vi "Chamber_control_Aug_ 2018.vi"() -> ()   [LabVIEW 2014]
doc: "This template is for the Queued Message Handler design pattern.\n\nThe Event Handling Loop generates messages based on user interface actions.\n\nThe Message Handling Loop processes messages generated by the Event Handling Loop, or by other messages. The messages are string values, so new messages can be added easily to the Message Cases case structure in the Message Handling Loop. Each message cluster can also provide an optional value for Message Data, which is a variant that can be converted to whatever message-specific data is required."
uses:
  <vilib>/Analysis/baseanly.llb/Mean (DBL).vi
  <vilib>/Instr/_visa.llb/VISA Configure Serial Port (Instr).vi
  Environmental Chamber LabVIEW and Instruments/Drivers and Software/Keithley 2100 Series/Public/Configure/Configure 2 Wire Resistance.vi
  <vilib>/Utility/file.llb/Read From Spreadsheet File (string).vi
  <vilib>/Utility/file.llb/Write To Spreadsheet File (string).vi
  Environmental Chamber LabVIEW and Instruments/Drivers and Software/LabVIEW 8.2 Drivers/keithley_24xx/Keithley 24XX/Public/Data/Read (Single Point).vi
  Environmental Chamber LabVIEW and Instruments/Drivers and Software/keithley_6430/Keithley 6430/Public/Data/Read (Single Point).vi
  Environmental Chamber LabVIEW and Instruments/Drivers and Software/keithley_6430/Keithley 6430/Keithley 6430.lvlib
  Environmental Chamber LabVIEW and Instruments/Drivers and Software/Keithley 2100 Series/Keithley 2100 Series.lvlib
  Environmental Chamber LabVIEW and Instruments/Drivers and Software/keithley_24xx/Keithley 24XX/Keithley 24XX.lvlib
  <vilib>/Analysis/NI_AALBase.lvlib
panel:
  in  "K2420 DC bias (V)":dbl=0.05
  in  "SYSTEM CONTROL":T1={"valve % open"=0.0, "Desired pressure"=0.0, "set Vapor sccm"=0.0, "set Gas sccm"=0.0, "Valve mode"=enum."% Open", "Pressure Mode"=enum."Abs. pressure", "analyte partial pressure"=23.8, "Actual"=0.0, "Read pressure (Torr)"=0.0, "Read vapor flow (sccm)"=0.0, "Read gas flow (sccm)"=0.0, "Save now"=FALSE, "Stop after seq."=TRUE, "Turbo pump\nauto on"=TRUE, "Integrate points"=0} caption="Pressure settings" {"Integrate points" min=0 max=100 step=1; "analyte partial pressure" min=0.0 max=100.0 step=5.0; "set Gas sccm" min=0 max=200 step=5; "set Vapor sccm" min=0 max=200 step=5; "Desired pressure" min=0.0 max=760.0 step=5.0; "valve % open" min=0.0 max=100.0 step=5.0 format="%#_2f"}
  in  "SAVE SAMPLE / ANALYTE NAMES":T2={"QCM1"="", "QCM2"="", "QCM3"="", "QCM4"="broken", "QCM5"="NOT WORKING", "QCM6"="", "SRS"="bareAu", "K-2420"="", "K-6430"="", "K-2100"="", "Gas"="NOT WORKING", "Vapor"="H2O", "Notes"=""} caption="Save samplffe names"
  in  "Clear all charts":bool
  out "K-6430":dbl(graph)
  out "K-2420":dbl(graph)
  out "File":path caption="DATA FILE"
  in  "Stop":bool
  out "QCM plot":T3(graph)
  out "K-2100":dbl(graph)
  out "State date/time":string caption="Program start time"
  out "J-KEM temp":dbl(graph)
  out "saving data?":bool
  out "pressure chart":dbl(graph)
  in  "SEQUENCE":T4 {"preview" items=["pressure", "gas flow", "vapor flow", "bias"]}
  # "100"
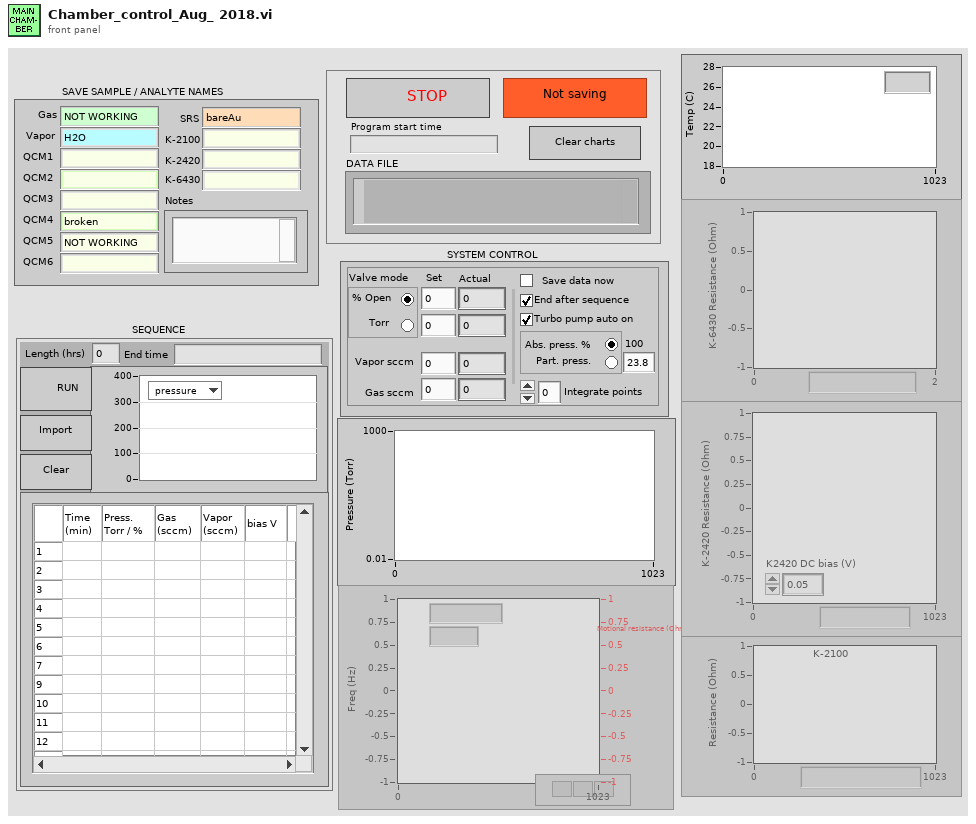
[diagram p1: front panel]
types:
  T1 = cluster{"valve % open":dbl, "Desired pressure":dbl, "set Vapor sccm":sgl, "set Gas sccm":sgl, "Valve mode":enum32{"% Open", "Torr "}, "Pressure Mode":enum32{"Abs. pressure", " Part. pressure"}, "analyte partial pressure":dbl, "Actual":dbl, "Read pressure (Torr)":dbl, "Read vapor flow (sccm)":dbl, "Read gas flow (sccm)":dbl, "Save now":bool, "Stop after seq.":bool, "Turbo pump\nauto on":bool, "Integrate points":i32}
  T2 = cluster{"QCM1":string, "QCM2":string, "QCM3":string, "QCM4":string, "QCM5":string, "QCM6":string, "SRS":string, "K-2420":string, "K-6430":string, "K-2100":string, "Gas":string, "Vapor":string, "Notes":string}
  T3 = cluster{"Frequency out":dbl, "Resistance out":dbl}
  T4 = cluster{"Run Sequence":bool, "User-defined\nsequence":string[][], "preview":u16, "Sequence\npreview":cluster{dbl[], dbl[]}[], "Clear sequence":bool, "Import sequence file":bool, "Length (hrs)":dbl, "End time":string}
  T5 = cluster{"Keithley 6430":bool, "J-KEM":bool, "Keithley 2420":bool, "Keithley 2100":bool, "SRS QCM":bool, "Pressure control":bool, "Arduino":bool}
  T6 = enum16{"open", "replace", "create", "open or create", "replace or create", "replace or create with confirmation"}
  T7 = enum8{"Enabled", "Disabled", "Disabled and Grayed Out"}
  T8 = cluster{"Frequency out":dbl, "Resistance out":dbl}[]
  T9 = cluster{"VISA resource name":refnum<visa-resource-name>, "error out":errorcluster, bool}
  T10 = cluster{"VISA resource name out":refnum<visa-resource-name>, "error out":errorcluster, bool}
  T11 = cluster{bool, "task out":refnum<k21>, "error out":errorcluster, "task out":refnum<k21>, "error out":errorcluster, "turbo pump":refnum<visa-resource-name>, "error out":errorcluster}
  T12 = cluster{bool, "task out":refnum<k21>, "error out":errorcluster, "task out":refnum<k21>, "error out":errorcluster, "VISA resource name out":refnum<visa-resource-name>, "error out":errorcluster}
  T13 = cluster{bool, "VISA resource name":refnum<visa-resource-name>, "error out":errorcluster}
  T14 = cluster{bool, "VISA resource name out":refnum<visa-resource-name>, "error out":errorcluster}
  T15 = cluster{bool, "VISA in":refnum<visa-resource-name>, "error out":errorcluster}
  T16 = cluster{bool, "VISA out":refnum<visa-resource-name>, "error out":errorcluster}
  T17 = cluster{"[0]":string, "[1]":string, "[2]":string, "[3]":string, "[4]":string, "[5]":string}
  T18 = cluster{string[][], path, "data headers":string[]}
  T19 = cluster{"Boolean":bool, "VISA resource name out":refnum<visa-resource-name>, "error out":errorcluster}
  T20 = cluster{"Boolean":bool, "VISA out":refnum<visa-resource-name>, "error out":errorcluster}
  T21 = cluster{cluster{bool, "VISA resource name out":refnum<visa-resource-name>, "error out":errorcluster}, "Address out":cluster{"Boolean":bool, "VISA resource name out":refnum<visa-resource-name>, "error out":errorcluster}, cluster{bool, "VISA resource name out":refnum<visa-resource-name>, "error out":errorcluster}, cluster{bool, "VISA resource name out":refnum<visa-resource-name>, "error out":errorcluster}, "SRS address out":cluster{"Boolean":bool, "VISA out":refnum<visa-resource-name>, "error out":errorcluster}}
  T22 = cluster{"valve % open":dbl, "Desired pressure":dbl, "set Vapor sccm":sgl, "set Gas sccm":sgl, "Valve mode":enum32{"% Open", "Torr "}, "Pressure Mode":enum32{"Abs. pressure", " Part. pressure"}, "analyte partial pressure":dbl}
  T23 = cluster{"User-defined\nsequence":string[][], "Present (s)":dbl, "current  step # in":i32, "sequence end time in":timestamp}
  T24 = cluster{"current  step # in":i32, "sequence end time in":timestamp, "Boolean":bool}
  T25 = cluster{"press/RH/gas/vapor":cluster{"pressure":string, "RH":string, "gas flow":string, "vapor flow":string}, "Cluster":cluster{"Valve position (%)":dbl, "read pressure":dbl, "read vapor flow":dbl, "read gas flow":dbl}}
  T26 = cluster{"Boolean":bool, "task out":refnum<k21>, "error out":errorcluster, "task out":refnum<k21>, "error out":errorcluster, "VISA resource name out":refnum<visa-resource-name>, "error out":errorcluster}
  T27 = cluster{"t":string, "delta t":string, "p":string, "delta p":string}
  T28 = cluster{"pressure":string, "RH":string, "gas flow":string, "vapor flow":string}
  T29 = cluster{"Valve position (%)":dbl, "read pressure":dbl, "read vapor flow":dbl, "read gas flow":dbl}
  T30 = cluster{"[0]":dbl, "[1]":dbl, "[2]":dbl, "[3]":dbl, "[4]":dbl, "[5]":dbl}[]
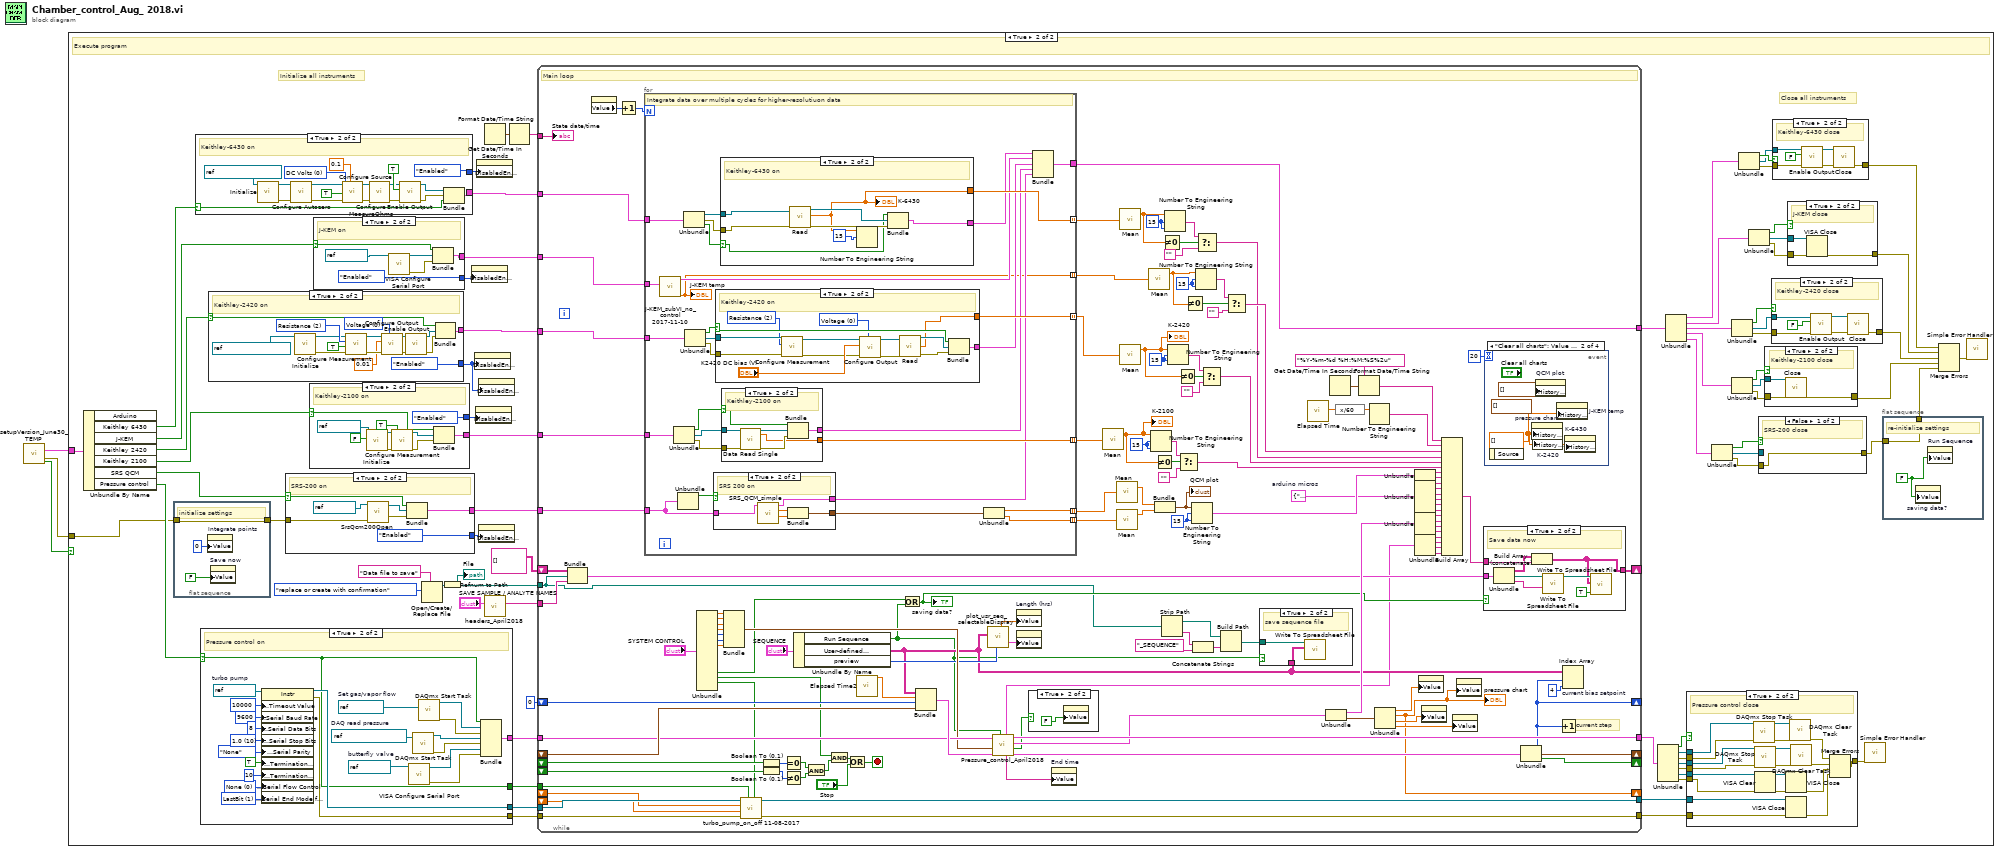
[diagram p0: block diagram]
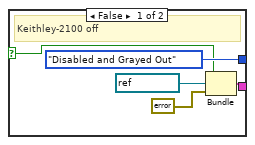
[diagram p4: hidden frame]
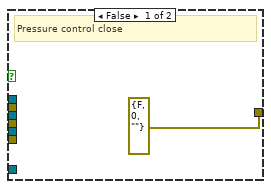
[diagram p5: hidden frame]
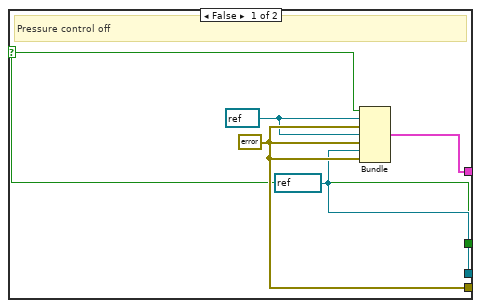
[diagram p6: hidden frame]
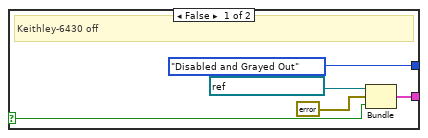
[diagram p8: hidden frame]
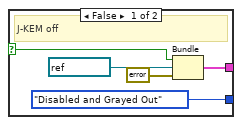
[diagram p10: hidden frame]
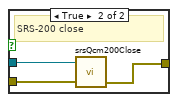
[diagram p11: hidden frame]
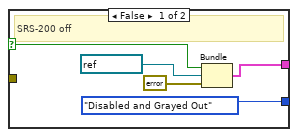
[diagram p12: hidden frame]
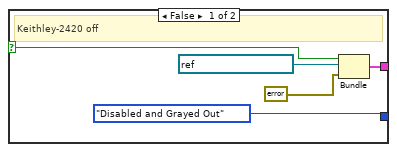
[diagram p14: hidden frame]
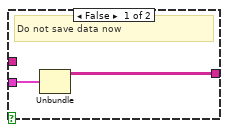
[diagram p16: hidden frame]
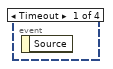
[diagram p17: hidden frame]
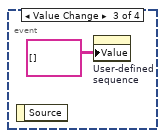
[diagram p18: hidden frame]
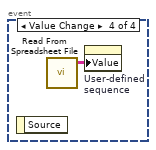
[diagram p19: hidden frame]
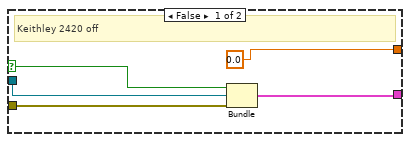
[diagram p20: hidden frame]
diagram:
  n1 = call "setupVersion_June30_TEMP.vi"() -> ("Instruments on/off"=w1:T5, "error IO"=w2:errorcluster, "OK"=w3:bool)  [unwired: 13 in]
  n2 = case shown="True" w3 {
    tunnel: w2 -> [_ w44]
    tunnel: w1 -> [_ w51]
    frame False {
      # "Cancel program"
    }
    frame True {
      # "Close all instruments"
      # "Initialize all instruments"
      # "Execute program"
      n3 = Unbundle By Name(w51) -> ("Keithley 6430"=w50:bool, "J-KEM"=w49:bool, "Keithley 2420"=w48:bool, "Keithley 2100"=w47:bool, "SRS QCM"=w46:bool, "Pressure control"=w45:bool)  [unwired: 1 out]
      n4 = flat-sequence {
        tunnel: [w78] -> w43
        tunnel: w44 -> [w78]
        frame #0 {
          # "initialize settings"
          n5 = property on="Integrate points" class="DigNum (strict)"("Value"=0) -> ()  [unwired: 2 in, 2 out]
          n6 = property on="Save now" class="Bool (strict)"("Value"=FALSE) -> ()  [unwired: 2 in, 2 out]
        }
      }
      n7 = case shown="True" w50 {
        selector: w50 -> [w156 w176]
        tunnel: [T7."Disabled and Grayed Out" ("Disabled") T7."Enabled" ("Disabled")] -> w30
        tunnel: [w155 w175] -> w28
        frame False {
          # "Keithley-6430 off"
          n8 = Bundle("VISA resource name"=refnum<visa-resource-name> "GPIB0::29::INSTR", "error out"=errorcluster {"status"=FALSE, "code"=0, "source"=""}, w156) -> (w155:T9)  [unwired: 1 in]
        }
        frame True {
          w163 = u16 0 items=["DC Volts", "DC Current"] ("Source Function (0: DC Volts)")
          # "Keithley-6430 on"
          n9 = call "Initialize.vi"("VISA resource name"=refnum<visa-resource-name> "GPIB2::19::INSTR") -> ("error out"=w169:errorcluster, "VISA resource name out"=w170:refnum<visa-resource-name>)  [unwired: 4 in, 5 out]
          n10 = call "Configure Autozero.vi"("error in (no error)"=w169, "VISA resource name"=w170) -> ("error out"=w166:errorcluster, "VISA resource name out"=w168:refnum<visa-resource-name>)  [unwired: 8 in]
          n11 = call "Configure Source.vi"("V-Source Level [V]"=0.1, "error in (no error)"=w166, "Auto Range (T:Enable)"=TRUE, "Source Function (0: DC Volts)"=w163, "VISA resource name"=w168) -> ("error out"=w165:errorcluster, "VISA resource name out"=w167:refnum<visa-resource-name>)  [unwired: 5 in]
          n12 = call "Configure MeasureOhms.vi"("error in (no error)"=w165, "VISA resource name"=w167) -> ("error out"=w174:errorcluster, "VISA resource name out"=w172:refnum<visa-resource-name>)  [unwired: 4 in, 4 out]
          n13 = call "Enable Output.vi"("error in (no error)"=w174, "Enable Output (F:Off)"=TRUE ("Output (F:Off)"), "VISA resource name"=w172) -> ("error out"=w161:errorcluster, "VISA resource name out"=w162:refnum<visa-resource-name>)  [unwired: 7 out]
          n14 = Bundle("VISA resource name out"=w162, "error out"=w161, w176) -> (w175:T10)  [unwired: 1 in]
        }
      }
      n15 = case shown="True" w45 {
        selector: w45 -> [w120 w126]
        tunnel: [w124 w127] -> w42
        tunnel: [w123 w125] -> w34
        tunnel: [w121 w128] -> w35
        tunnel: [w120 w126] -> w33
        frame False {
          w121 = refnum<visa-resource-name> refnum ("turbo pump")
          w122 = refnum<k21> refnum ("task out")
          w123 = errorcluster {"status"=FALSE, "code"=0, "source"=""} ("error out")
          # "Pressure control off"
          n16 = Bundle(w120, "task out"=w122, "error out"=w123, "task out"=w122, "error out"=w123, "turbo pump"=w121, "error out"=w123) -> (w124:T11)  [unwired: 1 in]
        }
        frame True {
          w132 = u16 1 items=["None", "LastBit", "TermChar"] ("Serial Settings:Serial End Mode for Reads")
          w130 = u16 0 items=["None", "XON/XOFF", "RTS/CTS", "XON/XOFF & RTS/CTS", "DTR/DSR", "XON/XOFF & DTR/DSR"] ("flow control (0:none)")
          w133 = u16 10 items=["1.0"=10, "1.5"=15, "2.0"=20] ("stop bits (10: 1 bit)")
          w129 = refnum<visa-resource-name> "COM7"  # turbo pump
          w145 = refnum<visa-resource-name> "COM5"  # butterfly valve
          w146 = refnum<k21> "Setflow"  # Set gas/vapor flow
          w147 = refnum<k21> "AllDaqReadings"  # DAQ read pressure
          # "Pressure control on"
          n17 = property class="Instr"(reference=w129, "General Settings:Timeout Value"=u32 10000 ("timeout (10sec)"), "Serial Settings:Serial Baud Rate"=u32 9600 ("baud rate (9600)"), "Serial Settings:Serial Data Bits"=u16 8 ("data bits (8)"), "Serial Settings:Serial Stop Bits"=w133, "Serial Settings:Serial Parity"=enum16{"None", "Odd", "Even", "Mark", "Space"}."None" ("parity (0:none)"), "Message Based Settings:Termination Character Enable"=TRUE ("Enable Termination\nChar (T)"), "Message Based Settings:Termination Character"=u8 10 ("termination char\n(0xA = '\\n' = LF)"), "Serial Settings:Serial Flow Control"=w130, "Serial Settings:Serial End Mode for Reads"=w132) -> (reference out=w128:refnum<visa-resource-name>, error out=w125:errorcluster)  [unwired: 1 in]
          n18 = call-poly "VISA Configure Serial Port"("VISA resource name"=w145) -> ("VISA resource name out"=w140:refnum<visa-resource-name>, "error out"=w139:errorcluster)  [unwired: 13 in]
          n19 = call <vilib>:"DAQmx Start Task.vi"("task/channels in"=w147) -> ("task out"=w142:refnum<k21>, "error out"=w141:errorcluster)  [unwired: 13 in]
          n20 = call <vilib>:"DAQmx Start Task.vi"("task/channels in"=w146) -> ("task out"=w144:refnum<k21>, "error out"=w143:errorcluster)  [unwired: 13 in]
          n21 = Bundle(w126, "task out"=w144, "error out"=w143, "task out"=w142, "error out"=w141, "VISA resource name out"=w140, "error out"=w139) -> (w127:T12)  [unwired: 1 in]
        }
      }
      n22 = case shown="True" w48 {
        selector: w48 -> [w219 w224]
        tunnel: [T7."Disabled and Grayed Out" ("Disabled") T7."Enabled" ("Disabled")] -> w17
        tunnel: [w217 w221] -> w27
        frame False {
          # "Keithley-2420 off"
          n23 = Bundle(w219, "VISA resource name"=refnum<visa-resource-name> "GPIB1::24::INSTR", "error out"=errorcluster {"status"=FALSE, "code"=0, "source"=""}) -> (w217:T13)  [unwired: 1 in]
        }
        frame True {
          w230 = u16 0 items=["Voltage", "Current"] ("Source Mode  (0: Voltage)")
          w235 = u16 2 items=["Volts", "Current", "Resistance"] ("Function (0: Volts)")
          # "Keithley-2420 on"
          n24 = call "Initialize.vi"("VISA resource name"=refnum<visa-resource-name> "GPIB1::24::INSTR") -> ("error out"=w225:errorcluster, "VISA resource name out"=w226:refnum<visa-resource-name>)  [unwired: 9 in]
          n25 = call "Configure Measurement.vi"("error in (no error)"=w225, "Enable Auto Range (T:Enable)"=TRUE, "Function (0: Volts)"=w235, "VISA resource name"=w226) -> ("error out"=w234:errorcluster, "VISA resource name out"=w233:refnum<visa-resource-name>)  [unwired: 6 in]
          n26 = call "Configure Output.vi"("Source Mode  (0: Voltage)"=w230, "error in (no error)"=w234, "Output Level (0)"=0.01 ("K2420 Applied Voltage (V) 2"), "VISA resource name"=w233) -> ("error out"=w232:errorcluster, "VISA resource name out"=w231:refnum<visa-resource-name>)  [unwired: 6 in]
          n27 = call "Enable Output.vi"("error in (no error)"=w232, "VISA resource name"=w231) -> ("error out"=w222:errorcluster, "VISA resource name out"=w223:refnum<visa-resource-name>)  [unwired: 8 in]
          n28 = Bundle(w224, "VISA resource name out"=w223, "error out"=w222) -> (w221:T14)  [unwired: 1 in]
        }
      }
      n29 = case shown="True" w46 {
        selector: w46 -> [w198 w204]
        tunnel: w43 -> [_ w207]
        tunnel: [T7."Disabled and Grayed Out" ("Disabled") T7."Enabled" ("Disabled")] -> w59
        tunnel: [w197 w203] -> w25
        frame False {
          # "SRS-200 off"
          n30 = Bundle(w198, "VISA in"=refnum<visa-resource-name> "COM6", "error out"=errorcluster {"status"=FALSE, "code"=0, "source"=""}) -> (w197:T15)  [unwired: 1 in]
        }
        frame True {
          # "SRS-200 on"
          n31 = call "SrsQcm200Open.vi"("error in"=w207, "VISA in"=refnum<visa-resource-name> "COM6") -> ("error out"=w202:errorcluster, "VISA out"=w205:refnum<visa-resource-name>)  [unwired: 3 in]
          n32 = Bundle(w204, "VISA out"=w205, "error out"=w202) -> (w203:T16)  [unwired: 1 in]
        }
      }
      n33 = case shown="True" w47 {
        selector: w47 -> [w88 w92]
        tunnel: [T7."Disabled and Grayed Out" ("Disabled") T7."Enabled" ("Disabled")] -> w57
        tunnel: [w85 w93] -> w26
        frame False {
          # "Keithley-2100 off"
          n34 = Bundle(w88, "VISA resource name out"=refnum<visa-resource-name> "K-2100", "error out"=errorcluster {"status"=FALSE, "code"=0, "source"=""}) -> (w85:T14)  [unwired: 1 in]
        }
        frame True {
          # "Keithley-2100 on"
          n35 = call "Initialize.vi"("VISA resource name"=refnum<visa-resource-name> "K-2100", "Reset? (T: Reset)"=FALSE) -> ("VISA resource name out"=w97:refnum<visa-resource-name>, "error out"=w96:errorcluster)  [unwired: 16 in]
          n36 = call-poly "Configure Measurement.vi"("VISA resource name"=w97, "error in (no error)"=w96, "Auto Range? (T: Auto)"=TRUE) -> ("VISA resource name out"=w91:refnum<visa-resource-name>, "error out"=w90:errorcluster)  [unwired: 15 in]
          n37 = Bundle(w92, "VISA resource name out"=w91, "error out"=w90) -> (w93:T14)  [unwired: 1 in]
        }
      }
      n38 = case shown="True" w49 {
        selector: w49 -> [w183 w189]
        tunnel: [w184 w190] -> w68
        tunnel: [T7."Disabled and Grayed Out" ("Disabled") T7."Enabled" ("Disabled")] -> w29
        frame False {
          # "J-KEM off"
          n39 = Bundle(w183, "VISA resource name"=refnum<visa-resource-name> "COM3", "error out"=errorcluster {"status"=FALSE, "code"=0, "source"=""}) -> (w184:T13)  [unwired: 1 in]
        }
        frame True {
          # "J-KEM on"
          n40 = call-poly "VISA Configure Serial Port"("VISA resource name"=refnum<visa-resource-name> "COM3") -> ("VISA resource name out"=w191:refnum<visa-resource-name>, "error out"=w188:errorcluster)  [unwired: 13 in]
          n41 = Bundle(w189, "VISA resource name out"=w191, "error out"=w188) -> (w190:T14)  [unwired: 1 in]
        }
      }
      n42 = Open/Create/Replace File(prompt="Data file to save", operation (0:open)=T6."replace or create with confirmation") -> (refnum out=w15:refnum<file>)  [unwired: 4 in, 2 out]
      n43 = Refnum to Path(1:w15) -> (0:w11:path)
      "File" <- w11
      n44 = property on="J-KEM temp" class="WFChart (strict)"("DisabledEnum"=w29) -> ()  [unwired: 2 in, 2 out]
      n45 = property on="K-2420" class="WFChart (strict)"("DisabledEnum"=w17) -> ()  [unwired: 2 in, 2 out]
      n46 = property on="K-2100" class="WFChart (strict)"("DisabledEnum"=w57) -> ()  [unwired: 2 in, 2 out]
      n47 = property on="K-6430" class="WFChart (strict)"("DisabledEnum"=w30) -> ()  [unwired: 2 in, 2 out]
      n48 = property on="K2420 DC bias (V)" class="DigNum (strict)"("DisabledEnum"=w17) -> ()  [unwired: 2 in, 2 out]
      n49 = property on="QCM plot" class="WFChart (strict)"("DisabledEnum"=w59) -> ()  [unwired: 2 in, 2 out]
      n50 = call "headers_April2018.vi"("Sample names"="SAVE SAMPLE / ANALYTE NAMES") -> ("data headers"=w10:string[])  [unwired: 10 in]
      n51 = Get Date/Time In Seconds() -> (seconds since 1Jan1904=w18:timestamp)
      n52 = Format Date/Time String(seconds (now)=w18) -> (date/time string=w56:string)  [unwired: 2 in]
      n53 = while {
        tunnel: w68 -> [w371]
        tunnel: w11 -> [w278]
        tunnel: w56 -> [w357]
        tunnel: w42 -> [w345]
        shift-right: [w332] -> _
        shift-left: 0 ("1st step") -> [w349]
        shift-right: [w354] -> _
        shift-left: _ -> [w352]
        shift-right: [w353] -> _
        shift-left: _ -> [w351]
        shift-left: _ -> [w350]
        tunnel: [w348] -> w53
        tunnel: w35 -> [w344]
        tunnel: w34 -> [w343]
        tunnel: w33 -> [w335]
        tunnel: [w341] -> w32
        tunnel: [w342] -> w31
        tunnel: w28 -> [w339]
        tunnel: w27 -> [w338]
        tunnel: w26 -> [w337]
        tunnel: w25 -> [w336]
        shift-right: [w291] -> _
        shift-left: _ -> [w334]
        shift-left: _ -> [w333]
        shift-right: [w288] -> _
        shift-left: string[][] [] -> [w286]
        tunnel: w10 -> [w285]
        tunnel: [w237] -> w9
        stop <- w363 stop-if-true
        w238 = T17 {"[0]"="", "[1]"="", "[2]"="", "[3]"="", "[4]"="", "[5]"=""}  # arduino micros
        w313 = i16 15 ("width (-)")
        w314 = i16 15 ("width (-)")
        w315 = i16 15 ("width (-)")
        w316 = i16 15 ("width (-)")
        w317 = i16 15 ("width (-)")
        # "current step"
        # "Main loop"
        n54 = Bundle(w286, w278, "data headers"=w285) -> (w282:T18)  [unwired: 1 in]
        n55 = property on="Integrate points" class="DigNum (strict)"() -> ("Value"=w284:i32)  [unwired: 2 in, 2 out]
        n56 = Increment(x=w284) -> (x+1=w319:i32)
        n57 = for {
          N: w319 -> [_]
          tunnel: w339 -> [w415]
          tunnel: w338 -> [w412]
          tunnel: w337 -> [w408]
          tunnel: w336 -> [w390]
          tunnel: w371 -> [w416]
          tunnel: [w403] -> w329 mode=indexing
          tunnel: [w402] -> w327 mode=indexing
          tunnel: [w389] -> w328 mode=indexing
          tunnel: [w401] -> w326 mode=indexing
          tunnel: [w399] -> w325 mode=indexing
          tunnel: [w398] -> w324 mode=indexing
          tunnel: [w392] -> w237
          # "Integrate data over multiple cycles for higher-resolutiuon data"
          n58 = call "J-KEM_subVI_no_control 2017-11-10.vi"("Address in"=w416) -> ("Temp (C)"=w389:dbl, "Address out"=w396:T19)  [unwired: 9 in]
          "J-KEM temp" <- w389
          n59 = Unbundle(w408) -> (w407:bool, "VISA resource name out"=w406:refnum<visa-resource-name>, "error out"=w405:errorcluster)
          n60 = Unbundle(w390) -> (w391:bool)  [unwired: 2 out]
          n61 = Unbundle(w415) -> ("VISA resource name out"=w414:refnum<visa-resource-name>, "error out"=w404:errorcluster, w413:bool)
          n62 = Unbundle(w412) -> (w411:bool, "VISA resource name out"=w410:refnum<visa-resource-name>, "error out"=w409:errorcluster)
          n63 = case "SRS QCM" shown="True" w391 {
            tunnel: [w461 w467] -> w393
            tunnel: [T3 {"Frequency out"=0.0, "Resistance out"=0.0} ("freq, MR") w464] -> w400
            tunnel: w390 -> [w461 w463]
            frame False {
              # "SRS QCM off"
            }
            frame True {
              # "SRS 200 on"
              n64 = call "SRS_QCM_simple.vi"("SRS address in"=w463) -> ("Resistance out"=w466:dbl, "Frequency out"=w465:dbl, "SRS address out"=w467:T20)  [unwired: 8 in]
              n65 = Bundle("Frequency out"=w465, "Resistance out"=w466) -> (w464:T3)  [unwired: 1 in]
            }
          }
          n66 = case shown="True" w411 {
            selector: w411 -> [w421 w435]
            tunnel: [w418 w434] -> w395
            tunnel: w410 -> [w420 w427]
            tunnel: w409 -> [w419 w425]
            tunnel: [sgl 0.0 ("Resistance") w422] -> w402
            frame False {
              # "Keithley 2420 off"
              n67 = Bundle(w421, "VISA resource name out"=w420, "error out"=w419) -> (w418:T14)  [unwired: 1 in]
            }
            frame True {
              w423 = u16 2 items=["Volts", "Current", "Resistance"] ("Function (0: Volts)")
              w431 = u16 0 items=["Voltage", "Current"] ("Source Mode  (0: Voltage)")
              # "Keithley-2420 on"
              n68 = call "Configure Measurement.vi"("error in (no error)"=w425, "Function (0: Volts)"=w423, "VISA resource name"=w427) -> ("error out"=w424:errorcluster, "VISA resource name out"=w426:refnum<visa-resource-name>)  [unwired: 7 in]
              n69 = call "Configure Output.vi"("Source Mode  (0: Voltage)"=w431, "error in (no error)"=w424, "Output Level (0)"="K2420 DC bias (V)", "VISA resource name"=w426) -> ("error out"=w429:errorcluster, "VISA resource name out"=w430:refnum<visa-resource-name>)  [unwired: 6 in]
              n70 = call-poly "Read.vi"("VISA resource name"=w430, "error in (no error)"=w429) -> ("VISA resource name out"=w433:refnum<visa-resource-name>, "Resistance"=w422:sgl, "error out"=w432:errorcluster)  [unwired: 7 in, 4 out]
              n71 = Bundle(w435, "VISA resource name out"=w433, "error out"=w432) -> (w434:T14)  [unwired: 1 in]
            }
          }
          n72 = case "Keithley 6430" shown="True" w413 {
            selector: w413 -> [w452 w455]
            tunnel: w414 -> [w451 w457]
            tunnel: [w450 w454] -> w397
            tunnel: w404 -> [w449 w456]
            tunnel: [0.0 ("K6340 Bias (V)") w453] -> w403
            frame False {
              # "Keithley-6430 off"
              n73 = Bundle(w452, "VISA resource name out"=w451, "error out"=w449) -> (w450:T14)  [unwired: 1 in]
            }
            frame True {
              # "Keithley-6430 on"
              n74 = call-poly "Read.vi"("error in (no error)"=w456, "VISA resource name"=w457) -> ("error out"=w458:errorcluster, "Measurement"=w453:dbl, "VISA resource name out"=w459:refnum<visa-resource-name>)  [unwired: 1 in, 6 out]
              "K-6430" <- w453
              n75 = Number To Engineering String(3:i16 15 ("width (-)"), 4:w453) -> ()  [unwired: 2 in, 1 out]
              n76 = Bundle(w455, "VISA resource name out"=w459, "error out"=w458) -> (w454:T14)  [unwired: 1 in]
            }
          }
          n77 = case shown="True" w407 {
            selector: w407 -> [w440 w445]
            tunnel: w406 -> [w438 w447]
            tunnel: w405 -> [w439 w446]
            tunnel: [w437 w442] -> w394
            tunnel: [0.0 ("Measurement") w441] -> w401
            frame False {
              # "Keithley-2100 off"
              n78 = Bundle(w440, "VISA resource name out"=w438, "error out"=w439) -> (w437:T14)  [unwired: 1 in]
            }
            frame True {
              # "Keithley-2100 on"
              n79 = call "Data Read Single.vi"("VISA resource name"=w447, "error in (no error)"=w446) -> ("VISA resource name out"=w444:refnum<visa-resource-name>, "Measurement"=w441:dbl, "error out"=w443:errorcluster)  [unwired: 15 in]
              n80 = Bundle(w445, "VISA resource name out"=w444, "error out"=w443) -> (w442:T14)  [unwired: 1 in]
            }
          }
          n81 = Unbundle(w400) -> ("Frequency out"=w399:dbl, "Resistance out"=w398:dbl)
          n82 = Bundle(w397, "Address out"=w396, w395, w394, "SRS address out"=w393) -> (w392:T21)  [unwired: 1 in]
        }
        n83 = Unbundle("SYSTEM CONTROL") -> ("valve % open"=w306:dbl, "Desired pressure"=w305:dbl, "set Vapor sccm"=w304:sgl, "set Gas sccm"=w303:sgl, "Valve mode"=w302:enum32{"% Open", "Torr "}, "Pressure Mode"=w301:enum32{"Abs. pressure", " Part. pressure"}, "analyte partial pressure"=w300:dbl, "Save now"=w294:bool, "Stop after seq."=w293:bool, "Turbo pump\nauto on"=w292:bool)  [unwired: 5 out]
        n84 = Bundle("valve % open"=w306, "Desired pressure"=w305, "set Vapor sccm"=w304, "set Gas sccm"=w303, "Valve mode"=w302, "Pressure Mode"=w301, "analyte partial pressure"=w300) -> (w307:T22)  [unwired: 1 in]
        n85 = call "turbo_pump_on_off 11-08-2017.vi"("Turbo pump\nauto on"=w292, "pressure control on?"=w335, "error in (no error)"=w343, "read pressure"=w333, "read pressure 2"=w334, "VISA Refnum in"=w344) -> ("error out"=w342:errorcluster, "VISA Refnum out"=w341:refnum<visa-resource-name>)  [unwired: 4 in]
        n86 = Boolean To (0,1)(Boolean=w351) -> (0, 1=w367:i16)
        n87 = Boolean To (0,1)(Boolean=w350) -> (0, 1=w366:i16)
        n88 = Equal To 0?(x=w367) -> (x = 0?=w364:bool)
        n89 = Not Equal To 0?(x=w366) -> (x != 0?=w365:bool)
        n90 = Unbundle By Name("SEQUENCE") -> ("Run Sequence"=w259:bool, "User-defined\nsequence"=w279:string[][], "preview"=w298:u16)
        n91 = And(x=w364, y=w365) -> (x .and. y?=w362:bool)
        n92 = And(x=w293, y=w362) -> (x .and. y?=w361:bool)
        n93 = Or(x=w361, y="Stop") -> (x .or. y?=w363:bool)
        n94 = call "Elapsed Time2"() -> ("Present (s)"=w312:dbl)  [unwired: 12 in, 7 out]
        n95 = Or(x=w294, y=w259) -> (x .or. y?=w287:bool)
        "saving data?" <- w287
        n96 = Bundle("User-defined\nsequence"=w279, "Present (s)"=w312, "current  step # in"=w349, "sequence end time in"=w352) -> (w356:T23)  [unwired: 1 in]
        n97 = call "plot_usr_seq_selectableDisplay.vi"("Display"=w298, "User-defined sequence"=w279) -> ("Sequence Preview"=w297:cluster{dbl[], dbl[]}[], "seq length (hours)"=w283:dbl)  [unwired: 8 in]
        n98 = call "Pressure_control_April2018.vi"("Run Sequence"=w259, "user sequence, present (s) in, current step in, seq time in"=w356, "pressure parameters in"=w307, "pressure control on?/daq IDs/errors"=w345) -> ("current step # out, shift register time out, seq button on?"=w355:T24, "sequence over? USE THIS TO REINITIALIZE RUN SEQUENCE BUTTON SO PROGRAM ENDS"=w296:bool, "save press/RH/gasflow/vaporflow - read valve position/pressure/vaporflow/gasflow"=w347:T25, "pressure control on?/daq IDs/errors out"=w348:T26, "sequence end date/time string"=w290:string, "abs_t, delta_t, abs_p, delta_p"=w264:T27)  [unwired: 2 in]
        n99 = property on="Length (hrs)" class="DigNum (strict)"("Value"=w283) -> ()  [unwired: 2 in, 2 out]
        n100 = property on="Sequence\npreview" class="XYGraph (strict)"("Value"=w297) -> ()  [unwired: 2 in, 2 out]
        n101 = case shown="True" w296 {
          frame False {
          }
          frame True {
            n102 = property on="Run Sequence" class="Bool (strict)"("Value"=FALSE ("Run Sequence")) -> ()  [unwired: 2 in, 2 out]
          }
        }
        n103 = property on="End time" class="Str"("Value"=w290) -> ()  [unwired: 2 in, 2 out]
        n104 = call-poly <vilib>:"Mean.vi"("X"=w326) -> ("mean"=w239:dbl)  [unwired: 1 out]
        "K-2100" <- w239
        n105 = call-poly <vilib>:"Mean.vi"("X"=w325) -> ("mean"=w323:dbl)  [unwired: 1 out]
        n106 = call-poly <vilib>:"Mean.vi"("X"=w324) -> ("mean"=w322:dbl)  [unwired: 1 out]
        n107 = call-poly <vilib>:"Mean.vi"("X"=w329) -> ("mean"=w246:dbl)  [unwired: 1 out]
        n108 = call-poly <vilib>:"Mean.vi"("X"=w327) -> ("mean"=w258:dbl)  [unwired: 1 out]
        "K-2420" <- w258
        n109 = call-poly <vilib>:"Mean.vi"("X"=w328) -> ("mean"=w251:dbl)  [unwired: 1 out]
        n110 = Number To Engineering String(2:w314, 3:w314, 4:w239) -> (0:w241:string)  [unwired: 1 in]
        n111 = Not Equal To 0?(x=w239) -> (x != 0?=w242:bool)
        n112 = Bundle("mean"=w323, "mean"=w322) -> (w321:cluster{"mean":dbl, "mean":dbl})  [unwired: 1 in]
        "QCM plot" <- w321
        n113 = Not Equal To 0?(x=w246) -> (x != 0?=w248:bool)
        n114 = Strip Path(path=w278) -> (stripped path=w281:path, name=w277:string)
        n115 = Number To Engineering String(2:w317, 3:w317, 4:w246) -> (0:w245:string)  [unwired: 1 in]
        n116 = Number To Engineering String(2:w315, 3:w315, 4:w258) -> (0:w256:string)  [unwired: 1 in]
        n117 = Not Equal To 0?(x=w258) -> (x != 0?=w257:bool)
        n118 = Select(t=w241, s=w242, f="") -> (s? t:f=w240:string)
        n119 = Not Equal To 0?(x=w251) -> (x != 0?=w252:bool)
        n120 = Number To Engineering String(2:w313, 3:w313, 4:w321) -> (0:w320:cluster{"mean":string, "mean":string})  [unwired: 1 in]
        n121 = Concatenate Strings(w277, "_SEQUENCE" ("name or relative path")) -> (w275:string)
        n122 = Number To Engineering String(2:w316, 3:w316, 4:w251) -> (0:w249:string)  [unwired: 1 in]
        n123 = Select(t=w245, s=w248, f="") -> (s? t:f=w244:string)
        n124 = Select(t=w256, s=w257, f="") -> (s? t:f=w255:string)
        n125 = Build Path(base path=w281, name or relative path=w275) -> (appended path=w280:path)
        n126 = Select(t=w249, s=w252, f="") -> (s? t:f=w250:string)
        n127 = case shown="True" w259 {
          tunnel: w280 -> [_ w374]
          tunnel: w279 -> [_ w373]
          frame False {
          }
          frame True {
            # "save sequence file"
            n128 = call-poly <vilib>:"Write To Spreadsheet File.vi"("2D data"=w373, "file path (dialog if empty)"=w374) -> ()  [unwired: 6 in, 1 out]
          }
        }
        n129 = call "Elapsed Time"() -> ("Elapsed Time (s)"=w330:dbl)  [unwired: 12 in, 7 out]
        n130 = Unbundle(w347) -> ("press/RH/gas/vapor"=w346:T28, "Cluster"=w311:T29)
        n131 = Get Date/Time In Seconds() -> (seconds since 1Jan1904=w372:timestamp)
        n132 = expression code="x/60"(w330) -> (w331:dbl)
        n133 = Format Date/Time String(time format string (%c)="%Y-%m-%d %H:%M:%S%2u", seconds (now)=w372) -> (date/time string=w368:string)  [unwired: 1 in]
        n134 = Number To Engineering String ("elapsed time (min)")(4:w331) -> (0:w358:string)  [unwired: 3 in]
        n135 = Unbundle(w311) -> ("Valve position (%)"=w310:dbl, "read pressure"=w291:dbl, "read vapor flow"=w309:dbl, "read gas flow"=w308:dbl)
        "pressure chart" <- w291
        n136 = Unbundle(w320) -> ("mean"=w359:string, "mean"=w369:string)
        n137 = Unbundle(w238) -> ("[0]"=w274:string, "[1]"=w273:string, "[2]"=w272:string, "[3]"=w271:string, "[4]"=w270:string, "[5]"=w269:string)
        n138 = Unbundle(w346) -> ("pressure"=w268:string, "RH"=w267:string, "gas flow"=w266:string, "vapor flow"=w265:string)
        n139 = Unbundle(w264) -> ("t"=w263:string, "delta t"=w262:string, "p"=w261:string, "delta p"=w260:string)
        n140 = property on="Actual" class="DigNum (strict)"("Value"=w310) -> ()  [unwired: 2 in, 2 out]
        n141 = property on="Read vapor flow (sccm)" class="DigNum (strict)"("Value"=w309) -> ()  [unwired: 2 in, 2 out]
        n142 = Build Array(w368, w358, w250, w244, w255, w240, w359, w369, w274, w273, w272, w271, w270, w269, w268, w267, w266, w265, w263, w262, w261, w260) -> (w289:string[])
        n143 = property on="Read gas flow (sccm)" class="DigNum (strict)"("Value"=w308) -> ()  [unwired: 2 in, 2 out]
        n144 = property on="Read pressure (Torr)" class="DigNum (strict)"("Value"=w291) -> ()  [unwired: 2 in, 2 out]
        n145 = case shown="True" w287 {
          tunnel: w289 -> [_ w384]
          tunnel: [w375 w381] -> w288
          tunnel: w282 -> [w376 w380]
          frame False {
            # "Do not save data now"
            n146 = Unbundle(w376) -> (w375:string[][])  [unwired: 2 out]
          }
          frame True {
            # "Save data now"
            n147 = Unbundle(w380) -> (w379:string[][], w378:path, "data headers"=w377:string[])
            n148 = Build Array (concatenate)(w379, w384) -> (w381:string[][])
            n149 = call-poly <vilib>:"Write To Spreadsheet File.vi"("1D data"=w377, "file path (dialog if empty)"=w378) -> ("new file path (Not A Path if cancelled)"=w382:path)  [unwired: 6 in]
            n150 = call-poly <vilib>:"Write To Spreadsheet File.vi"("append to file? (new file:F)"=TRUE, "2D data"=w381, "file path (dialog if empty)"=w382) -> ()  [unwired: 5 in, 1 out]
          }
        }
        n151 = event shown="[1] \"Clear all charts\": Value Change" {
          selector: _ -> [_ _ _ _]
          dyn-events: _ -> [_ _ _ _]
          timeout: 20 -> [_ _ _ _]
          event Timeout {
            n152 = event-data() -> ()  [unwired: 1 in, 1 out]
          }
          event "Clear all charts": Value Change {
            (unwired) T30 [] ("History Data")
            w385 = dbl[] [] ("History Data")
            n153 = event-data() -> ()  [unwired: 1 in, 1 out]
            n154 = property on="pressure chart" class="WFChart (strict)"("History Data"=w385) -> ()  [unwired: 2 in, 2 out]
            n155 = property on="K-2420" class="WFChart (strict)"("History Data"=w385) -> ()  [unwired: 2 in, 2 out]
            n156 = property on="QCM plot" class="WFChart (strict)"("History Data"=T8 []) -> ()  [unwired: 2 in, 2 out]
            n157 = property on="J-KEM temp" class="WFChart (strict)"("History Data"=w385) -> ()  [unwired: 2 in, 2 out]
            n158 = property on="K-6430" class="WFChart (strict)"("History Data"=w385) -> ()  [unwired: 2 in, 2 out]
          }
          event "SEQUENCE.Clear sequence": Value Change {
            n159 = event-data() -> ()  [unwired: 1 in, 1 out]
            n160 = property on="User-defined\nsequence" class="Tbl (strict)"("Value"=string[][] []) -> ()  [unwired: 2 in, 2 out]
          }
          event "SEQUENCE.Import sequence file": Value Change {
            n161 = event-data() -> ()  [unwired: 1 in, 1 out]
            n162 = call-poly <vilib>:"Read From Spreadsheet File.vi"() -> ("all rows"=w388:string[][])  [unwired: 7 in, 4 out]
            n163 = property on="User-defined\nsequence" class="Tbl (strict)"("Value"=w388) -> ()  [unwired: 2 in, 2 out]
          }
        }
        n164 = Unbundle(w355) -> ("current  step # in"=w332:i32, "sequence end time in"=w354:timestamp, "Boolean"=w353:bool)
        n165 = Increment(x=w332) -> ()  [unwired: 1 out]
        n166 = Index Array "current bias setpoint"(array=w279, index (row)=w332, index (col)=4 ("disabled index (col)")) -> ()  [unwired: 1 out]
        "State date/time" <- w357
      }
      n167 = Unbundle(w53) -> ("Boolean"=w52:bool, "task out"=w41:refnum<k21>, "error out"=w40:errorcluster, "task out"=w39:refnum<k21>, "error out"=w38:errorcluster, "VISA resource name out"=w37:refnum<visa-resource-name>, "error out"=w36:errorcluster)
      n168 = Unbundle(w9) -> (w8:T14, "Address out"=w7:T19, w6:T14, w5:T14, "SRS address out"=w4:T20)
      n169 = case shown="True" w52 {
        tunnel: [errorcluster {"status"=FALSE, "code"=0, "source"=""} ("error out") w111] -> w55
        tunnel: w41 -> [_ w110]
        tunnel: w40 -> [_ w109]
        tunnel: w39 -> [_ w108]
        tunnel: w38 -> [_ w105]
        tunnel: w37 -> [_ w106]
        tunnel: w36 -> [_ w107]
        tunnel: w32 -> [_ w102]
        tunnel: w31 -> [_ w101]
        frame False {
          # "Pressure control close"
        }
        frame True {
          # "Pressure control close"
          n170 = call <vilib>:"DAQmx Stop Task.vi"("task/channels in"=w110, "error in"=w109) -> ("task out"=w117:refnum<k21>, "error out"=w116:errorcluster)  [unwired: 12 in]
          n171 = call <vilib>:"DAQmx Stop Task.vi"("task/channels in"=w108, "error in"=w105) -> ("task out"=w118:refnum<k21>, "error out"=w119:errorcluster)  [unwired: 12 in]
          n172 = VISA Clear(VISA resource name=w106, error in (no error)=w107) -> (VISA resource name out=w115:refnum<visa-resource-name>, error out=w114:errorcluster)
          n173 = VISA Close(VISA resource name=w102, error in (no error)=w101) -> (error out=w103:errorcluster)
          n174 = VISA Close(VISA resource name=w115, error in (no error)=w114) -> (error out=w104:errorcluster)
          n175 = call <vilib>:"DAQmx Clear Task.vi"("task in"=w117, "error in"=w116) -> ("error out"=w113:errorcluster)  [unwired: 13 in]
          n176 = call <vilib>:"DAQmx Clear Task.vi"("task in"=w118, "error in"=w119) -> ("error out"=w112:errorcluster)  [unwired: 13 in]
          n177 = Merge Errors(w113, w112, w104, w103) -> (w111:errorcluster)
        }
      }
      n178 = Unbundle(w4) -> ("Boolean"=w70:bool, "VISA out"=w69:refnum<visa-resource-name>, "error out"=w21:errorcluster)
      n179 = Unbundle(w6) -> (w73:bool, "VISA resource name out"=w72:refnum<visa-resource-name>, "error out"=w71:errorcluster)
      n180 = Unbundle(w5) -> (w24:bool, "VISA resource name out"=w23:refnum<visa-resource-name>, "error out"=w22:errorcluster)
      n181 = Unbundle(w8) -> (w63:bool, "VISA resource name out"=w62:refnum<visa-resource-name>, "error out"=w61:errorcluster)
      n182 = Unbundle(w7) -> ("Boolean"=w67:bool, "VISA resource name out"=w66:refnum<visa-resource-name>, "error out"=w65:errorcluster)
      n183 = case shown="False" w70 {
        tunnel: [w193 w196] -> w20
        tunnel: w69 -> [_ w195]
        tunnel: w21 -> [w193 w194]
        frame False {
          # "SRS-200 close"
        }
        frame True {
          # "SRS-200 close"
          n184 = call "srsQcm200Close.vi"("error in"=w194, "Visa in"=w195) -> ("error out"=w196:errorcluster)  [unwired: 3 in]
        }
      }
      n185 = case shown="True" w24 {
        tunnel: w23 -> [_ w84]
        tunnel: w22 -> [w81 w83]
        tunnel: [w81 w82] -> w58
        frame False {
          # "Keithley-2100 close"
        }
        frame True {
          # "Keithley-2100 close"
          n186 = call "Close.vi"("VISA resource name"=w84, "error in (no error)"=w83) -> ("error out"=w82:errorcluster)  [unwired: 17 in]
        }
      }
      n187 = case shown="True" w73 {
        tunnel: w72 -> [_ w212]
        tunnel: w71 -> [w209 w211]
        tunnel: [w209 w210] -> w74
        frame False {
          # "Keithley-2420 close"
        }
        frame True {
          # "Keithley-2420 close"
          n188 = call "Enable Output.vi"("error in (no error)"=w211, "Enable Output (T: Enable)"=FALSE, "VISA resource name"=w212) -> ("error out"=w213:errorcluster, "VISA resource name out"=w215:refnum<visa-resource-name>)  [unwired: 7 in]
          n189 = call "Close.vi"("error in (no error)"=w213, "VISA resource name"=w215) -> ("error out"=w210:errorcluster)  [unwired: 9 in]
        }
      }
      n190 = case shown="True" w63 {
        tunnel: w62 -> [_ w150]
        tunnel: w61 -> [w148 w149]
        tunnel: [w148 w151] -> w60
        frame False {
          # "Keithley-6430 close"
        }
        frame True {
          # "Keithley-6430 close"
          n191 = call "Enable Output.vi"("error in (no error)"=w149, "Enable Output (F:Off)"=FALSE ("Output (F:Off)"), "VISA resource name"=w150) -> ("error out"=w152:errorcluster, "VISA resource name out"=w153:refnum<visa-resource-name>)  [unwired: 7 out]
          n192 = call "Close.vi"("error in (no error)"=w152, "VISA resource name"=w153) -> ("error out"=w151:errorcluster)  [unwired: 9 out]
        }
      }
      n193 = case shown="True" w67 {
        tunnel: w66 -> [_ w181]
        tunnel: w65 -> [w178 w180]
        tunnel: [w178 w179] -> w64
        frame False {
          # "J-KEM close"
        }
        frame True {
          # "J-KEM close"
          n194 = VISA Close(VISA resource name=w181, error in (no error)=w180) -> (error out=w179:errorcluster)
        }
      }
      n195 = call <vilib>:"Simple Error Handler.vi"("error in (no error)"=w55) -> ()  [unwired: 4 in, 5 out]
      n196 = flat-sequence {
        tunnel: w20 -> [w80]
        tunnel: [w80] -> w19
        frame #0 {
          w79 = FALSE ("saving data?")
          # "re-initialize settings"
          n197 = property on="saving data?" class="Bool (strict)"("Value"=w79) -> ()  [unwired: 2 in, 2 out]
          n198 = property on="Run Sequence" class="Bool (strict)"("Value"=w79) -> ()  [unwired: 2 in, 2 out]
        }
      }
      n199 = Merge Errors(w60, w64, w74, w58, w19) -> (w75:errorcluster)
      n200 = call <vilib>:"Simple Error Handler.vi"("error in (no error)"=w75) -> ()  [unwired: 4 in, 5 out]
    }
  }
